vi "updateUnits.vi"(8 "error in (no error)":errorcluster, 11 "ActionEditor in":refnum<class "ActionEditor.lvclass">) -> (0 "error out":errorcluster, 3 "ActionEditor out":refnum<class "ActionEditor.lvclass">)   [LabVIEW 2009, in "Views.lvlib" / "ScriptEditor.lvlib" / "ActionEditor.lvclass"]
uses:
  ActionEditor.lvclass
  ActionEditor.lvclass/ActionEditor.ctl
  Tools/Scripting/ScriptingEvent/ScriptEvent.lvclass
  Tools/DatabaseHelpers/Database Objects/Channel/Channel.lvclass
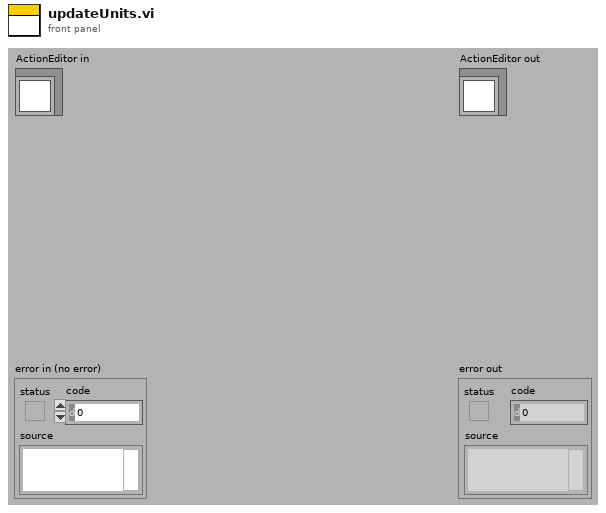
[diagram p1: front panel]
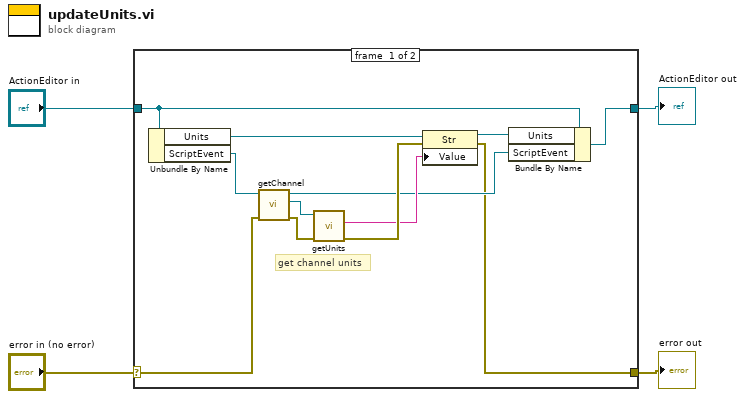
[diagram p0: block diagram]
diagram:
  n1 = case shown="No Error" "error in (no error)" {
    selector: "error in (no error)" -> [w13 w18]
    tunnel: [w7 w18] -> w3
    tunnel: [w5 w17] -> w1
    tunnel: "ActionEditor in" -> [w6 w17]
    frame #0 {
      # "get channel units"
      n2 = Unbundle By Name(w6) -> ("Units"=w12:refnum<vi>, "ScriptEvent"=w16:refnum<class "ScriptEvent.lvclass">)
      n3 = call-dynamic "getChannel.vi"("error in (no error)"=w13, "ScriptEvent.lvclass in"=w16) -> ("error out"=w14:errorcluster, "Channel.lvclass"=w15:refnum<class "Channel.lvclass">, "ScriptEvent.lvclass out"=w8:refnum<class "ScriptEvent.lvclass">)  [unwired: 7 in]
      n4 = call-dynamic "getUnits.vi"("error in (no error)"=w14, "Channel.lvclass in"=w15) -> ("error out"=w11:errorcluster, "units"=w10:string)  [unwired: 7 in, 1 out]
      n5 = property class="Str"(reference=w12, error in=w11, "Value"=w10) -> (reference out=w9:refnum<vi>, error out=w7:errorcluster)
      n6 = Bundle By Name(cluster=w6, "Units"=w9, "ScriptEvent"=w8) -> (w5:refnum<class "ActionEditor.lvclass">)
    }
    frame #1 {
    }
  }
  "error out" <- w3
  "ActionEditor out" <- w1
